vi "mic_filter.vi"() -> ()   [LabVIEW 2020]
uses:
  <vilib>/ptbypt/NI_PtbyPt.lvlib
panel:
  out "Time has Elapsed":bool
  out "Amplitude 2":dbl
  out "Amplitude":dynamicdata(graph)
  in  "stop":bool
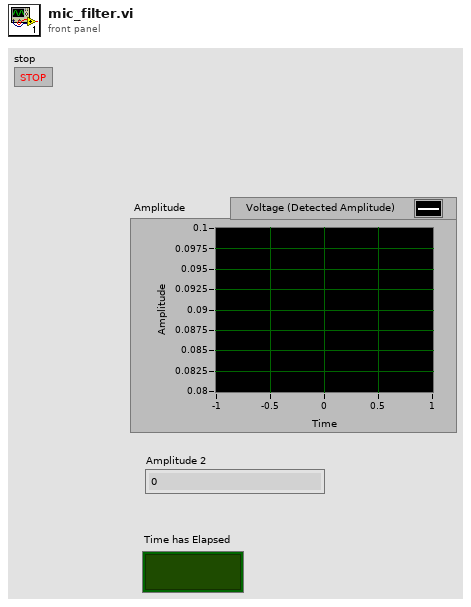
[diagram p1: front panel]
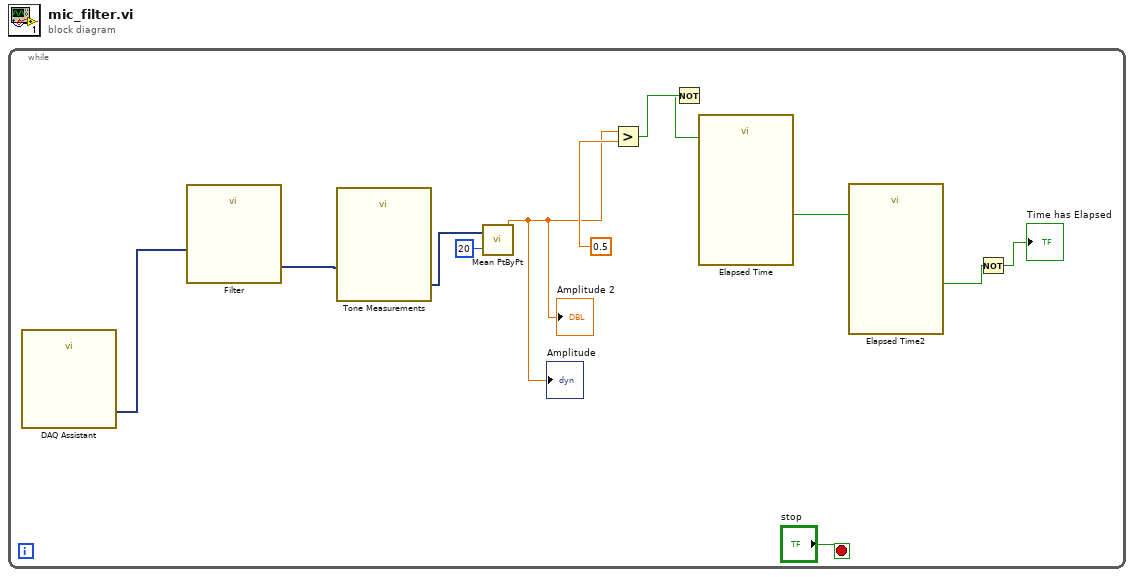
[diagram p0: block diagram]
diagram:
  n1 = while {
    stop <- "stop" stop-if-true
    n2 = call "DAQ Assistant"() -> ("data"=w7:dynamicdata)  [unwired: 17 in, 2 out]
    n3 = call "Filter"("Signal"=w7) -> ("Filtered Signal"=w12:dynamicdata)  [unwired: 9 in, 1 out]
    n4 = call "Tone Measurements"("Signals"=w12) -> ("Amplitude"=w6:dynamicdata)  [unwired: 9 in, 1 out]
    n5 = call <vilib>:"Mean PtByPt.vi"("x"=w6, "sample length"=20) -> ("mean"=w4:dbl)  [unwired: 2 in, 1 out]
    "Amplitude" <- w4
    "Amplitude 2" <- w4
    n6 = Greater?(x=w4, y=0.5) -> (0:w10:bool)
    n7 = Not(x=w10) -> (.not. x?=w9:bool)
    n8 = call "Elapsed Time"("Reset"=w9) -> ("Time has Elapsed"=w3:bool)  [unwired: 11 in, 7 out]
    n9 = call "Elapsed Time2"("Reset"=w3) -> ("Time has Elapsed"=w2:bool)  [unwired: 11 in, 7 out]
    n10 = Not(x=w2) -> (.not. x?=→"Time has Elapsed":bool)
  }
